vi "Upload values to ADAM server.vi"() -> ()   [LabVIEW 2022 SP3]
uses:
  Anemometry Sub Vis/Controls/Save_Data.ctl
  Anemometry Sub Vis/Controls/Setup.ctl
  Anemometry Sub Vis/Controls/Post_Process.ctl
  Anemometry Sub Vis/Globals/Meas_global.vi
panel:
  in  "Averaging time (min)":dbl=1.0 format="%.2f"
  in  "stop":bool
  in  "Results file":path=path "C:/Enflo_Data_Local/2019/Laser_Disp_Scanner/Lam Chan/Results/Res_01-2019/Wind_Turbine_Displacement2.xls"
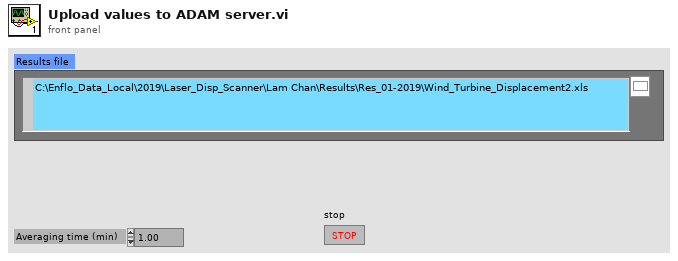
[diagram p1: front panel]
types:
  T1 = typedef "Post_Process.ctl" = enum16{"Take New Data", "Post Process Raw Data File"}
  T2 = typedef "Setup.ctl" = enum16{"Run Program", "Show Setup", "Save Current Setup", "Setup Front Panel"}
  T3 = typedef "Save_Data.ctl" = enum16{"Save No Data", "Save Data"}
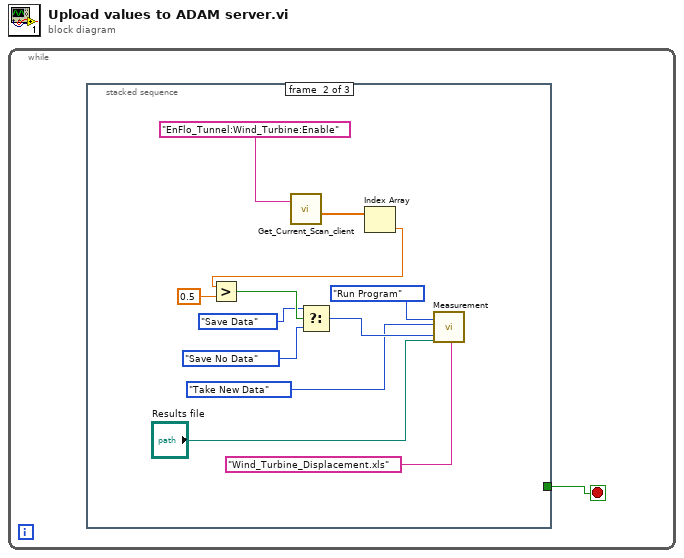
[diagram p0: block diagram]
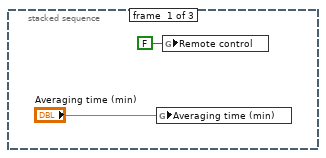
[diagram p2: hidden frame]
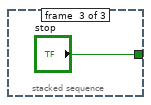
[diagram p3: hidden frame]
diagram:
  n1 = while {
    stop <- w1 stop-if-true
    n2 = stacked-sequence {
      tunnel: [_ _ "stop"] -> w1
      frame #0 {
        n3 = global write "Meas_global.vi" "Averaging time (min)"("Averaging time (min)") -> ()
        n4 = global write "Meas_global.vi" "Remote control"(FALSE ("Remote control")) -> ()
      }
      frame #1 {
        n5 = call "Get_Current_Scan_client.vi"("singleChannel"="EnFlo_Tunnel:Wind_Turbine:Enable") -> ("Numerical Values"=w15:dbl[])  [unwired: 1 in, 3 out]
        n6 = Index Array(array=w15) -> (element=w14:dbl)  [unwired: 1 in]
        n7 = Greater?(x=w14, y=0.5) -> (0:w12:bool)
        n8 = Select(t=Save_Data."Save Data" ("File"), s=w12, f=Save_Data."Save No Data" ("File")) -> (s? t:f=w9:T3)
        n9 = call "Measurement.vi"("setup"=Setup."Run Program", "Post Process"=Post_Process."Take New Data", "File"=w9, "Results file"="Results file", "Setup filename"="Wind_Turbine_Displacement.xls") -> ()  [unwired: 13 in, 2 out]
      }
      frame #2 {
      }
    }
  }
